vi "Read TCS parameters.vi"(8 "error in (no error)":errorcluster, 11 "TCS_ACS in":refnum<class "TCS_ACS.lvclass">) -> (0 "error out":errorcluster, 2 "TCS parameters":T1, 3 "TCS_ACS out":refnum<class "TCS_ACS.lvclass">)   [LabVIEW 2018, in "TCS_ACS.lvclass"]
uses:
  TCS_ACS.lvclass
  TCS_ACS.lvclass/TCS_ACS.ctl
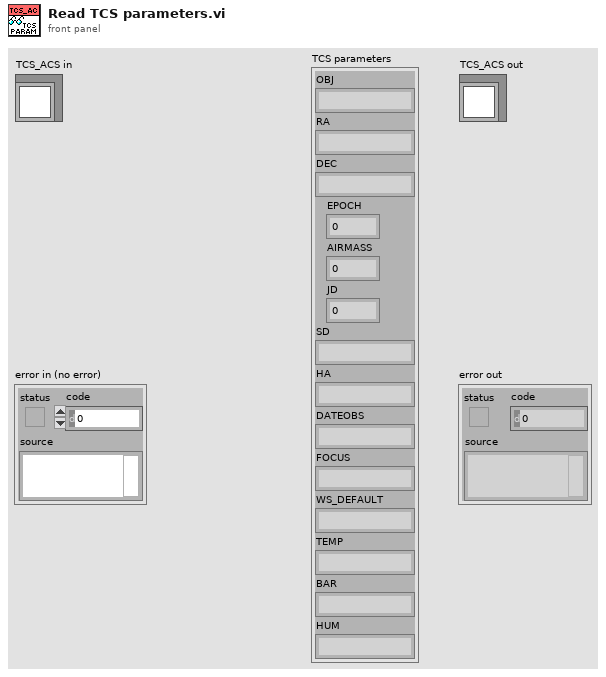
[diagram p1: front panel]
types:
  T1 = cluster{"OBJ":string, "RA":string, "DEC":string, "EPOCH":dbl, "AIRMASS":dbl, "JD":dbl, "SD":string, "HA":string, "DATEOBS":string, "FOCUS":string, "WS_DEFAULT":string, "TEMP":string, "BAR":string, "HUM":string}
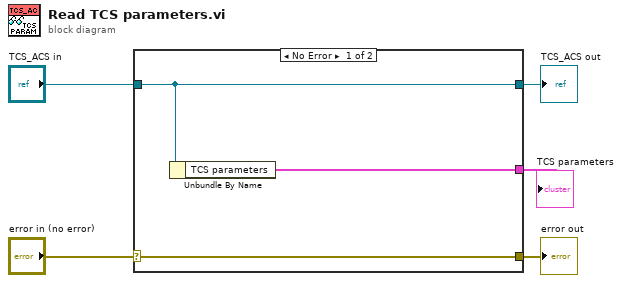
[diagram p0: block diagram]
diagram:
  n1 = case shown="No Error" "error in (no error)" {
    selector: "error in (no error)" -> [w8 w9]
    tunnel: [w8 w9] -> w4
    tunnel: [w7 w10] -> w2
    tunnel: "TCS_ACS in" -> [w7 w10]
    tunnel: [w6 _] -> w1
    frame No Error {
      n2 = Unbundle By Name(w7) -> ("TCS parameters"=w6:T1)
    }
    frame Error {
    }
  }
  "error out" <- w4
  "TCS_ACS out" <- w2
  "TCS parameters" <- w1
